vi "000 Display Format.vi"(11 "Data":T1) -> (3 "Data":string[](array[string]))   [LabVIEW 2020]
uses:
  Global/Data Global/SDQ Data Type.ctl
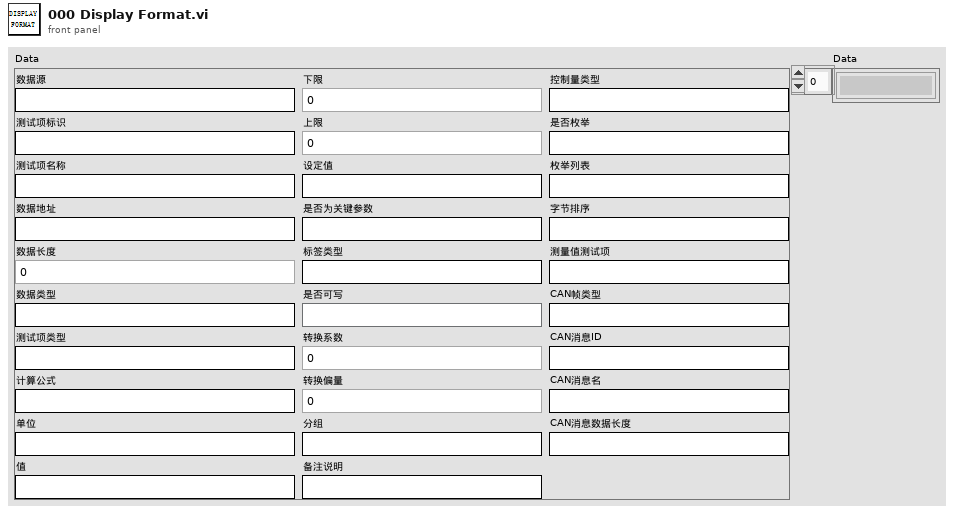
[diagram p1: front panel]
types:
  T1 = typedef "SDQ Data Type.ctl" = cluster{"CAN Length":string, "CAN Name":string, "CAN ID":string, "CAN Type":string, "Test Item":string, "Byte Order":string, "Instruction":string, "Control Type":string, "Group":string, "Offset":dbl, "Coefficient":dbl, "Write Enable":bool, "Lable Type":string, "Key?":string, "Set Value":string, "Upper":dbl, "Lower":dbl, "Unit":string, "Formula":string, "Test Item Type":string, "Length":i32, "Address":string, "Name":string, "Identifier":string, "Data Type":string, "Enumerate?":string, "Enumerate List":string, "Data":string, "Source":string}
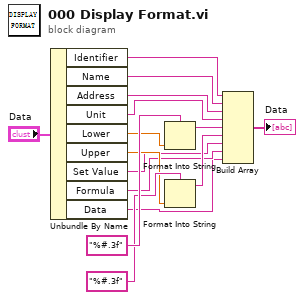
[diagram p0: block diagram]
diagram:
  n1 = Unbundle By Name("Data") -> ("Identifier"=w4:string, "Name"=w1:string, "Address"=w15:string, "Unit"=w14:string, "Lower"=w12:dbl, "Upper"=w9:dbl, "Set Value"=w7:string, "Formula"=w6:string, "Data"=w5:string)
  n2 = Format Into String(format string="%#.3f" ("格式字符串"), w12) -> (resulting string=w11:string)  [unwired: 2 in, 1 out]
  n3 = Format Into String(format string="%#.3f" ("格式字符串"), w9) -> (resulting string=w8:string)  [unwired: 2 in, 1 out]
  n4 = Build Array(w4, w1, w15, w14, w11, w8, w7, w6, w5) -> (→"Data":string[])
